vi "Preflight Time Series.vi"(8 "error in":errorcluster, 10 "Exp params":T1={"Experiment Type"="Time Series", "Experiment Name"="qwerty2", "ExpPath"=path "E:/test", "Save As"="TDMS", "TSFrames"=100, "TSfps"=50.0, "Streaming"=FALSE, "tdms ref"=refnum, "frame #"=0, "Full Path"=path "E:/test/qwerty2", "PeakOnQueue"=FALSE} {"TSFrames" min=1 step=1; "TSfps" min=0.001 max=90.0 step=0.001 format="%_4g"}, 11 "Camera Controls":T3={"Exposure Time (ms)"=27, "cam0 Session"="cam0", "Camera ROI"={"Width"=1100, "Height"=600, "Offset X"=0, "Offset Y"=0}, "Command"=""} {"Camera ROI"."Offset Y" max=2046 step=2; "Camera ROI"."Offset X" max=2044 step=4; "Camera ROI"."Height" min=2 max=2048 step=2; "Camera ROI"."Width" min=4 max=2048 step=4; "Exposure Time (ms)" min=27 max=500 step=1 scale=27.0..500.0}) -> (0 "error out":errorcluster, 2 "Exp params out":T1={"Experiment Type"="Time Series", "Experiment Name"="qwerty2", "ExpPath"=path "E:/test", "Save As"="TDMS", "TSFrames"=100, "TSfps"=10.0, "Streaming"=FALSE, "tdms ref"=refnum, "frame #"=0, "Full Path"=path "E:/test/qwerty2", "PeakOnQueue"=FALSE} {"TSFrames" min=1 step=1; "TSfps" min=0.001 max=90.0 step=0.001 format="%_4g"}, 3 "CamSession out":T2="cam0")   [LabVIEW 2020]
uses:
  _controls/xiCam.ctl
  <vilib>/userDefined/High Color/IMAQdx.ctl
  _controls/Exp Params.ctl
  _controls/Timer_actions.ctl
  <vilib>/vision/driver/NI_Vision_Acquisition_Software.lvlib
  <resource>/objmgr/imaqdx.rc
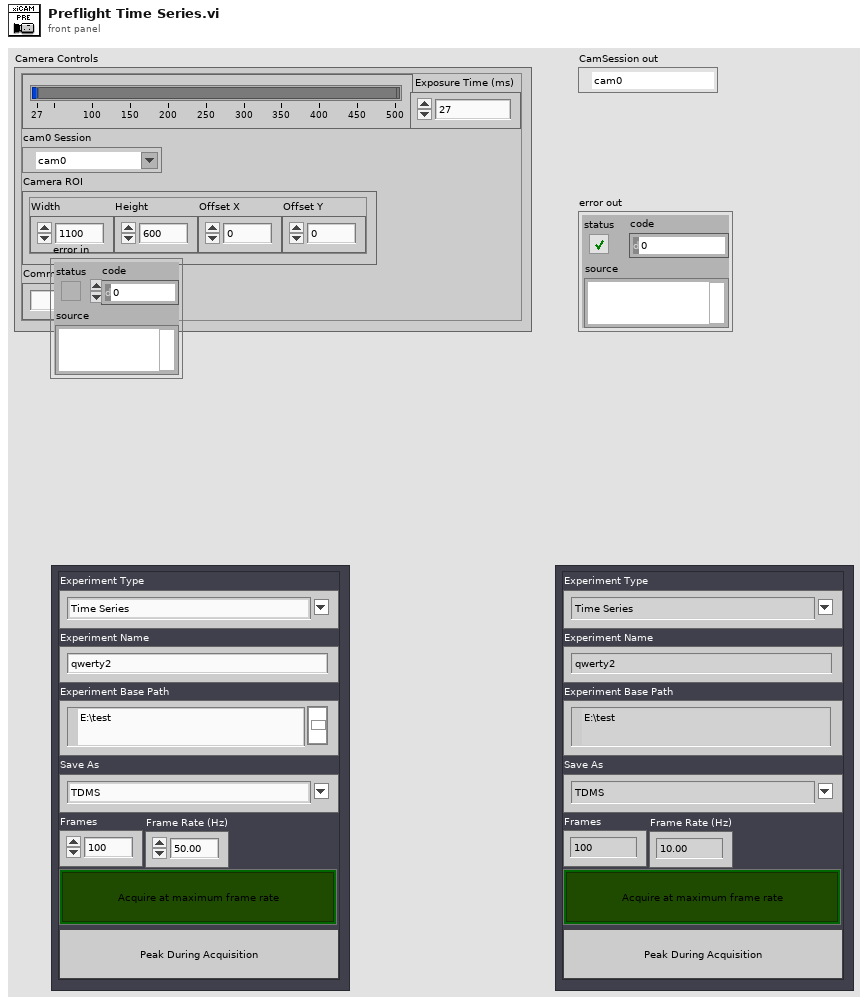
[diagram p1: front panel]
types:
  T1 = typedef "Exp Params.ctl" = cluster{"Experiment Type":string, "Experiment Name":string, "ExpPath":path, "Save As":string, "TSFrames":i32, "TSfps":dbl, "Streaming":bool, "tdms ref":refnum<k34>, "frame #":i64, "Full Path":path, "PeakOnQueue":bool}
  T2 = typedef "IMAQdx.ctl" = refnum<k21>
  T3 = typedef "xiCam.ctl" = cluster{"Exposure Time (ms)":u32, "cam0 Session":T2, "Camera ROI":cluster{"Width":u32, "Height":u32, "Offset X":u32, "Offset Y":u32}, "Command":string}
  T4 = typedef "Timer_actions.ctl" = enum16{"Reset", "Snap", "Total"}
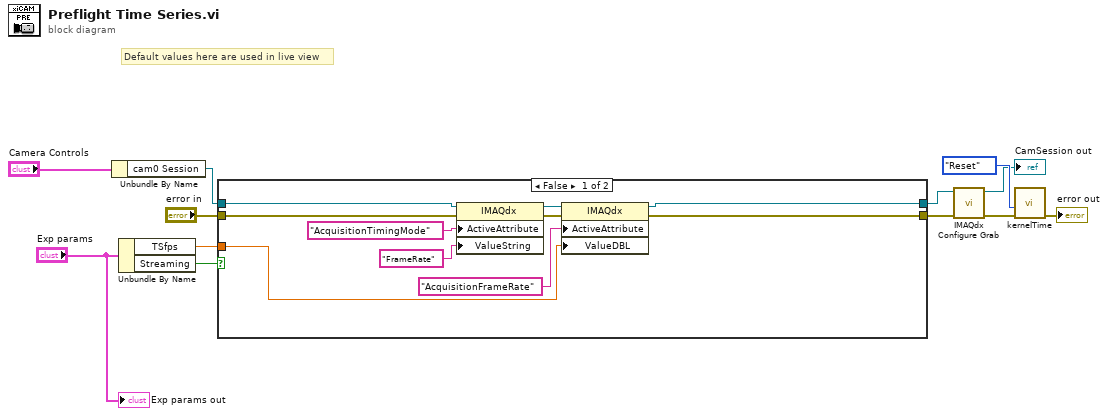
[diagram p0: block diagram]
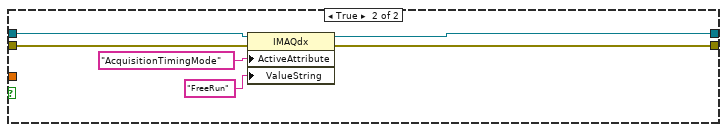
[diagram p2: hidden frame]
diagram:
  # "Default values here are used in live view"
  n1 = Unbundle By Name("Camera Controls") -> ("cam0 Session"=w7:T2)
  n2 = Unbundle By Name("Exp params") -> ("TSfps"=w2:dbl, "Streaming"=w1:bool)
  n3 = case shown="False" w1 {
    tunnel: w7 -> [w16 w26]
    tunnel: "error in" -> [w15 w25]
    tunnel: w2 -> [w21 _]
    tunnel: [w20 w24] -> w5
    tunnel: [w19 w23] -> w4
    frame False {
      n4 = property class="IMAQdx"(reference=w16, error in=w15, "ActiveAttribute"="AcquisitionTimingMode", "ValueString"="FrameRate") -> (reference out=w13:T2, error out=w14:errorcluster)
      n5 = property class="IMAQdx"(reference=w13, error in=w14, "ActiveAttribute"="AcquisitionFrameRate", "ValueDBL"=w21) -> (reference out=w20:T2, error out=w19:errorcluster)
    }
    frame True {
      n6 = property class="IMAQdx"(reference=w26, error in=w25, "ActiveAttribute"="AcquisitionTimingMode", "ValueString"="FreeRun") -> (reference out=w24:T2, error out=w23:errorcluster)
    }
  }
  n7 = call <vilib>:"IMAQdx Configure Grab.vi"("error in"=w4, "Session In"=w5) -> ("error out"=w10:errorcluster, "Session Out"=→"CamSession out":T2)  [unwired: 8 in]
  n8 = call "kernelTime.vi"("error in (no error) in"=w10, "Action (Snap)"=Timer_actions."Reset") -> ("error out"=→"error out":errorcluster)  [unwired: 8 in, 1 out]
  "Exp params out" <- "Exp params"
